vi "Lookapp.vi"(6 "App Name":string="My Application", 8 "error in":errorcluster, 11 "reference":refnum<vi>) -> (0 "error out":errorcluster, 3 "Project Item Ref":refnum<vi>)   [LabVIEW 2021, in "App-Builder Library.lvlib" / "Builder.lvclass"]
uses:
  Builder.lvclass
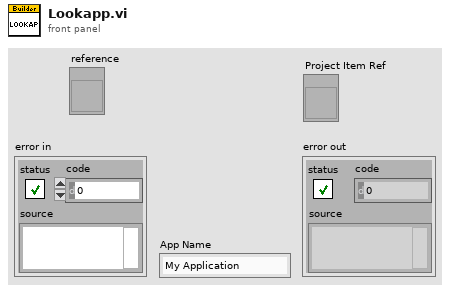
[diagram p1: front panel]
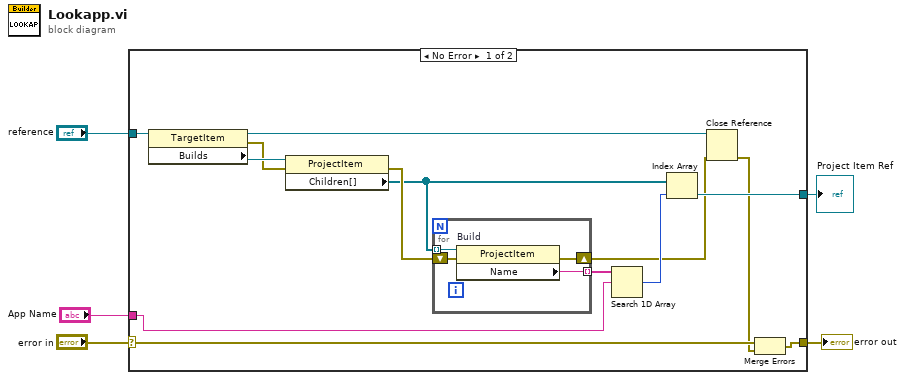
[diagram p0: block diagram]
diagram:
  n1 = case shown="No Error" "error in" {
    selector: "error in" -> [w19 w24]
    tunnel: [w7 w24] -> w4
    tunnel: "reference" -> [w13 _]
    tunnel: "App Name" -> [w12 _]
    tunnel: [w11 _] -> w1
    frame No Error {
      n2 = property class="TargetItem"(reference=w13) -> (reference out=w9:refnum<vi>, error out=w10:errorcluster, "Builds"=w18:refnum<vi>)  [unwired: 1 in]
      n3 = property class="ProjectItem"(reference=w18, error in=w10) -> (error out=w15:errorcluster, "Children[]"=w14:refnum<vi>[])  [unwired: 1 out]
      n4 = for {
        tunnel: w14 -> [w23] mode=indexing
        tunnel: [w22] -> w17 mode=indexing
        shift-right: [w20] -> w8
        shift-left: w15 -> [w21]
        n5 = property on="Build" class="ProjectItem"(reference=w23, error in=w21) -> (error out=w20:errorcluster, "Name"=w22:string)  [unwired: 1 out]
      }
      n6 = Search 1D Array(1D array=w17, element=w12) -> (index of element=w16:i32)  [unwired: 1 in]
      n7 = Index Array(array=w14, index=w16) -> (element=w11:refnum<vi>)
      n8 = Close Reference(reference=w9, error in (no error)=w8) -> (error out=w6:errorcluster)
      n9 = Merge Errors(w19, w6) -> (w7:errorcluster)
    }
    frame Error {
    }
  }
  "error out" <- w4
  "Project Item Ref" <- w1
